vi "PROCESS_CREATION_SCRIPTING.vi"() -> ()   [LabVIEW 2011]
uses:
  Ctl/ClusterDefineNewProcess.ctl
  050 - CONFIG/20 - ExternalProcesses/paramsExternalProcesses.ctl
  Ctl/AppContext.ctl
  Ctl/EnumProcessState.ctl
  Ctl/ClusterProcessCreationScript.ctl
  Ctl/EnumFPOrder.ctl
  <vilib>/event_ctls.llb/eventvkey.ctl
  <vilib>/regexp/Match Regular Expression.xnode
panel:
  in  "discardKey":bool
  in  "Cluster_process":T1={"Process name"="", "viToLaunchInfos"={"File Path Control"=path "", "Timeout"=10.0, "viInitString"="", "State"=enum."Standard"}}
  out "error out":errorcluster
  in  "Test PushButton":bool
  in  "Delete Process PushButton":bool
  in  "Existing processes":i32(listbox)
  in  "Close PushButton":bool
  in  "Create Process PushButton":bool
  # "PROCESS CREATION WIZARD"
  # "Version 1.0"
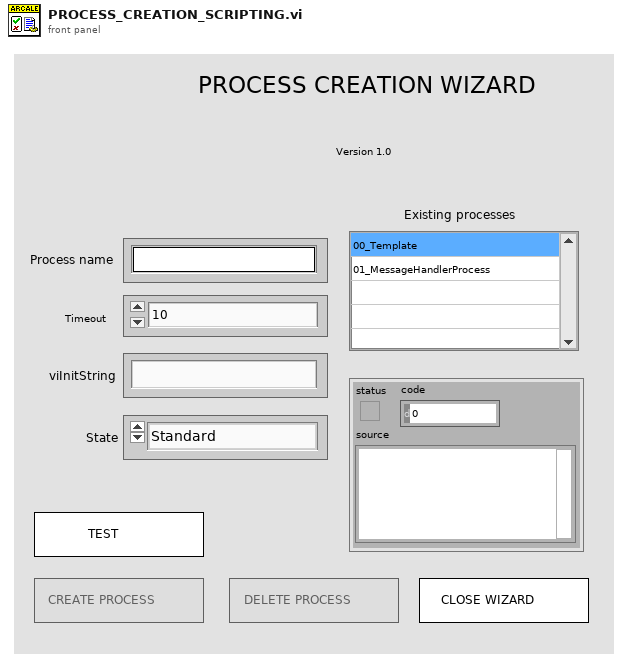
[diagram p1: front panel]
types:
  T1 = typedef "ClusterDefineNewProcess.ctl" = cluster{"Process name":string, "viToLaunchInfos":T2}
  T2 = typedef "paramsExternalProcesses.ctl" = cluster{"File Path Control":path, "Timeout":dbl, "viInitString":string, "State":enum32{"Invalid", "Standard", "Closed", "Hidden", "Minimized", "Maximized"}}
  T3 = enum8{"Enabled", "Disabled", "Disabled and Grayed Out"}
  T4 = typedef "AppContext.ctl" = cluster{"VIRefToProcessTemplate":refnum<vi>, "VIRefToThisVI":refnum<vi>, "ProcessesList":string[], "VIRefToEnumProcess":refnum<vi>, "VIRefTogetProcessViPath":refnum<vi>, "ProcessManagement":cluster{"EnumProcessState":T5, "ProcessName":string, "PathToProcess":path}, "VIRefToSetup":refnum<vi>, "VIRefToStartProcess":refnum<vi>, "ProcessConfig":T2}
  T5 = typedef "EnumProcessState.ctl" = enum16{"Create process", "Delete process"}
  T6 = typedef "ClusterProcessCreationScript.ctl" = cluster{"Variant":variant, "Front Panel Order":T7}
  T7 = typedef "EnumFPOrder.ctl" = enum16{"Test", "Create process", "Delete process", "Close wizard"}
  T8 = typedef "eventvkey.ctl" = enum16{"ASCII", "Enter", "Return", "Shift", "Ctrl", "Alt", "Cmd", "Opt", "Caps", "NumLock", "Clear", "Break", "Up", "Down", "Left", "Right", "Insert", "Delete", "Home", "End", "PageUp", "PageDown", "Escape", "Help", "Pause", "ScrollLock", "F1", "F2", "F3", "F4", "F5", "F6", "F7", "F8", "F9", "F10", "F11", "F12", "F13", "F14", "F15", "F16", "F17", "F18", "F19", "F20", "F21", "F22", "F23", "F24", "Play", "VolumeUp", "VolumeDown", "Mute", "Two Byte Char"}
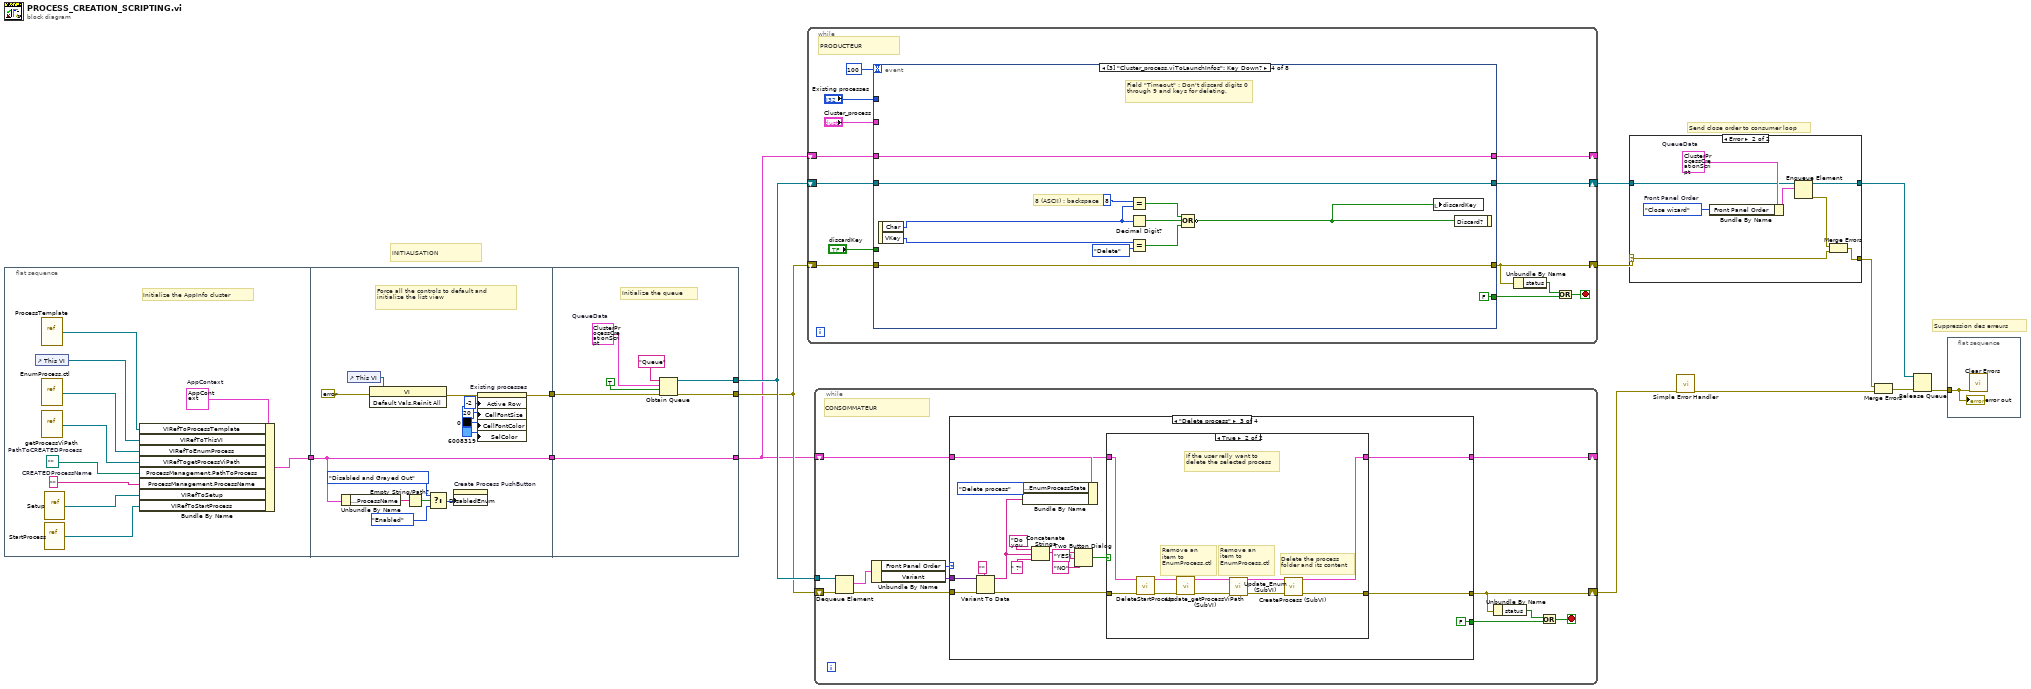
[diagram p0: block diagram]
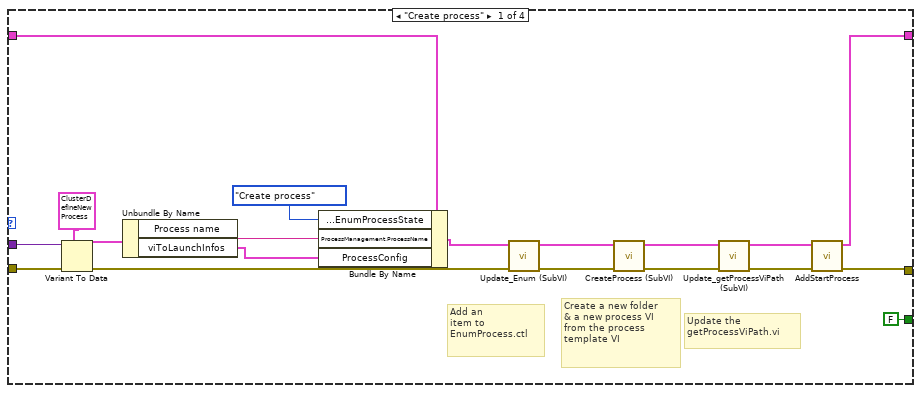
[diagram p3: hidden frame]
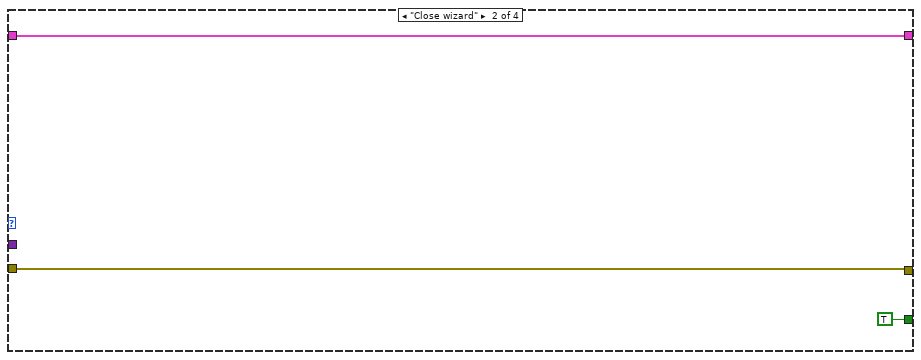
[diagram p4: hidden frame]
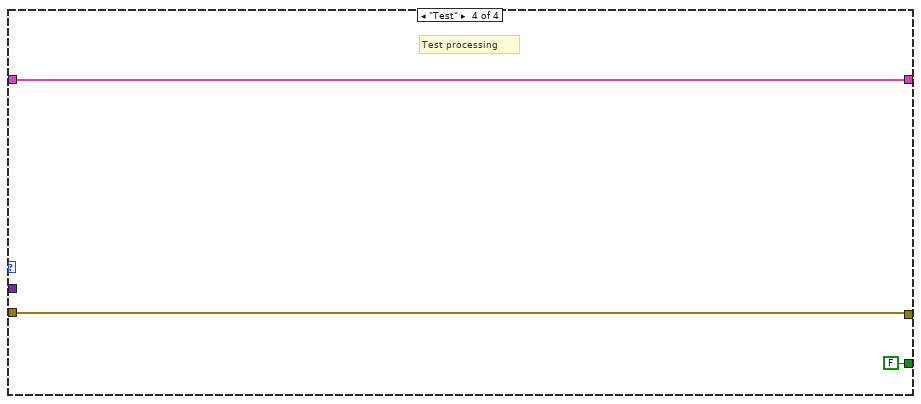
[diagram p6: hidden frame]
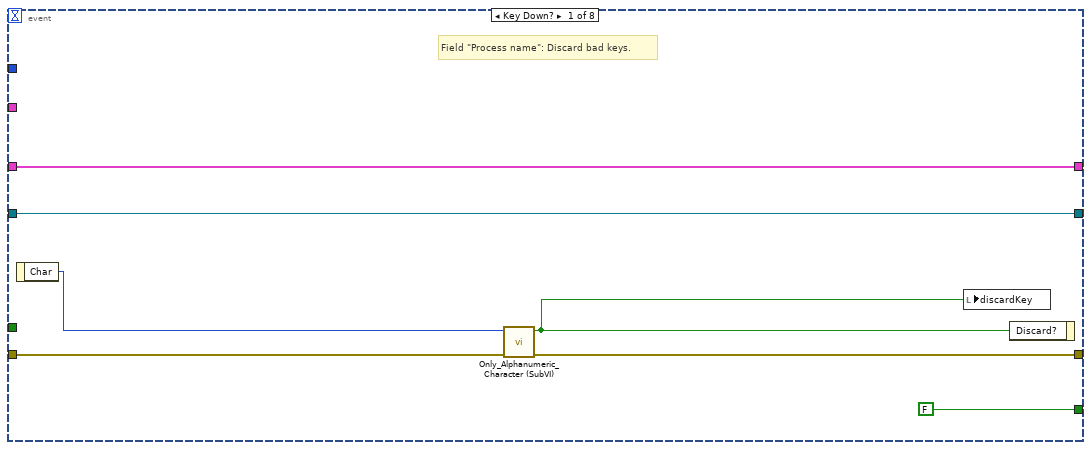
[diagram p7: hidden frame]
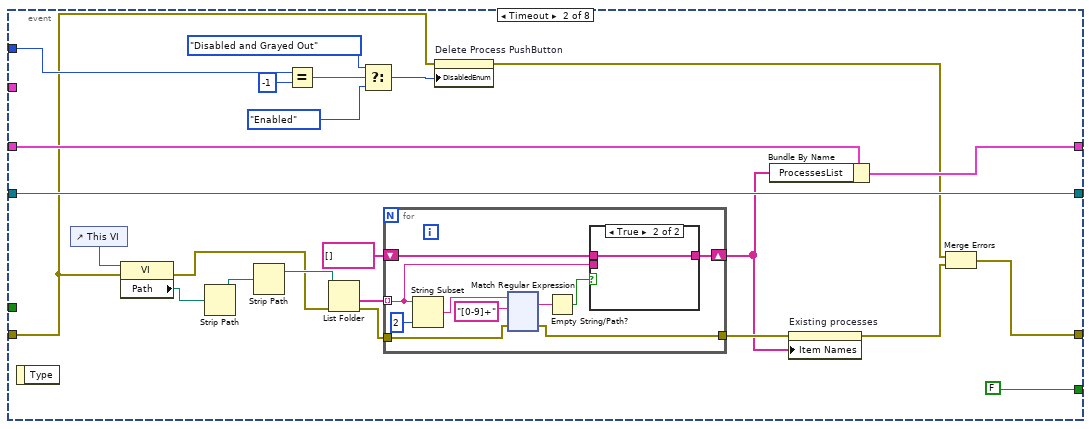
[diagram p8: hidden frame]
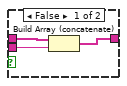
[diagram p9: hidden frame]
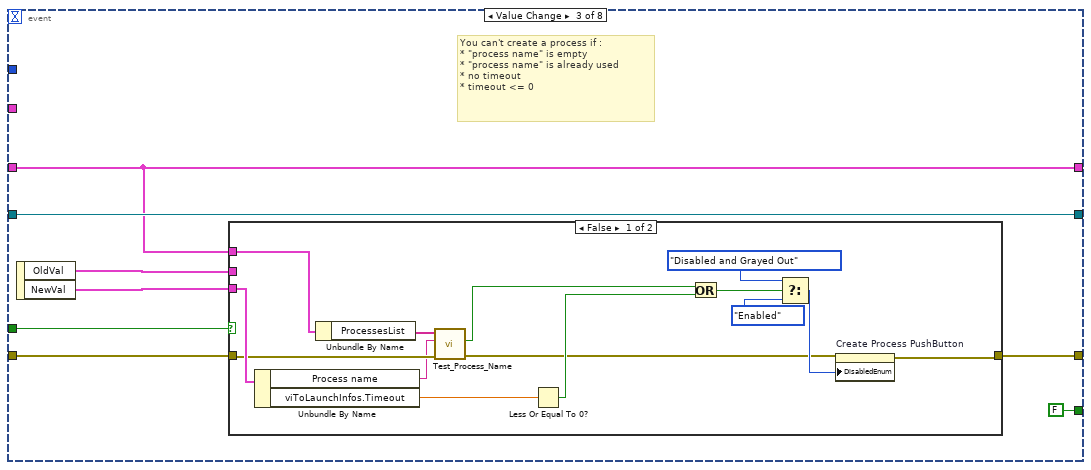
[diagram p10: hidden frame]
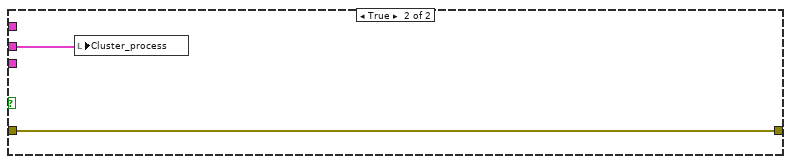
[diagram p11: hidden frame]
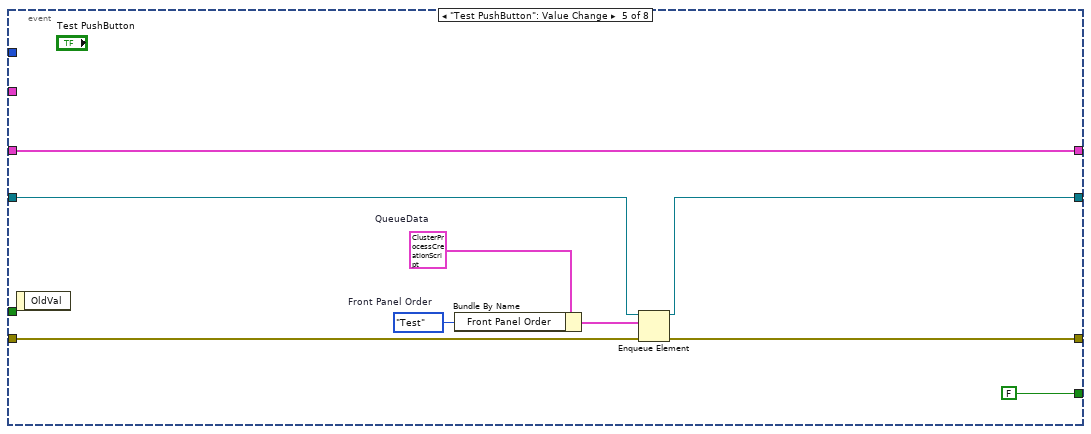
[diagram p12: hidden frame]
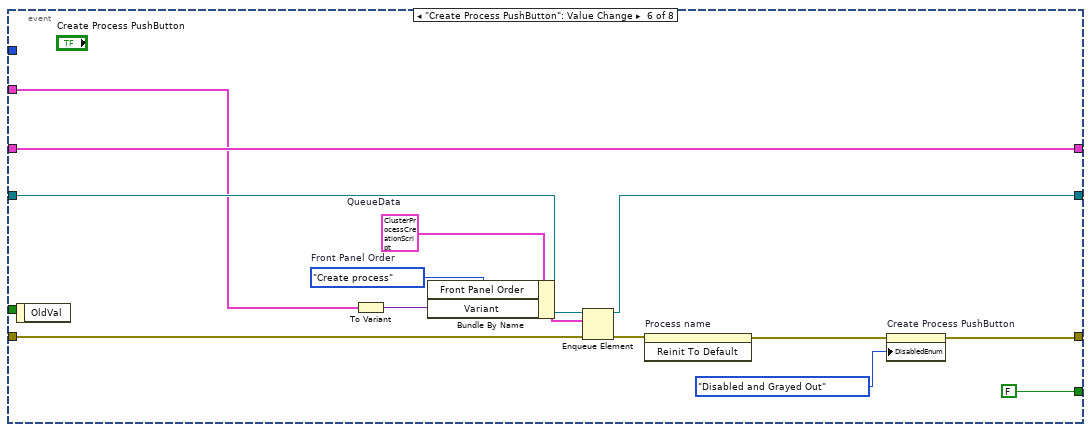
[diagram p13: hidden frame]
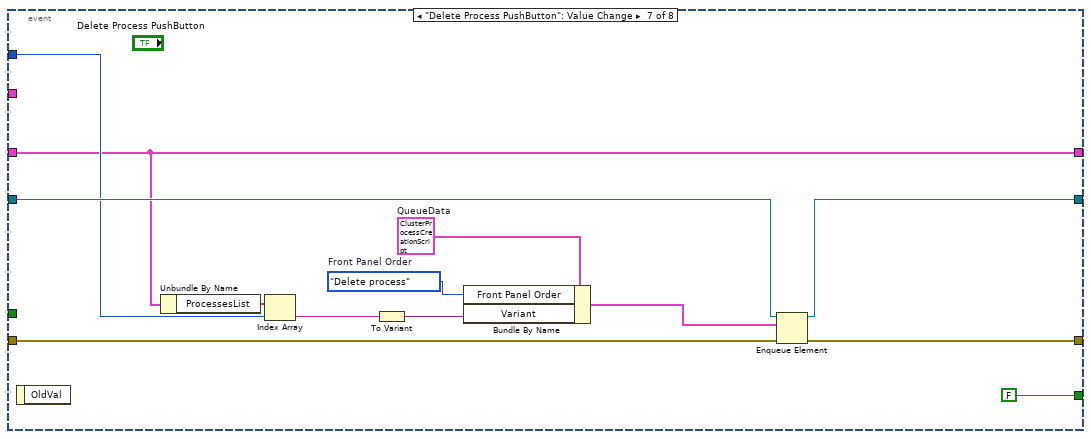
[diagram p14: hidden frame]
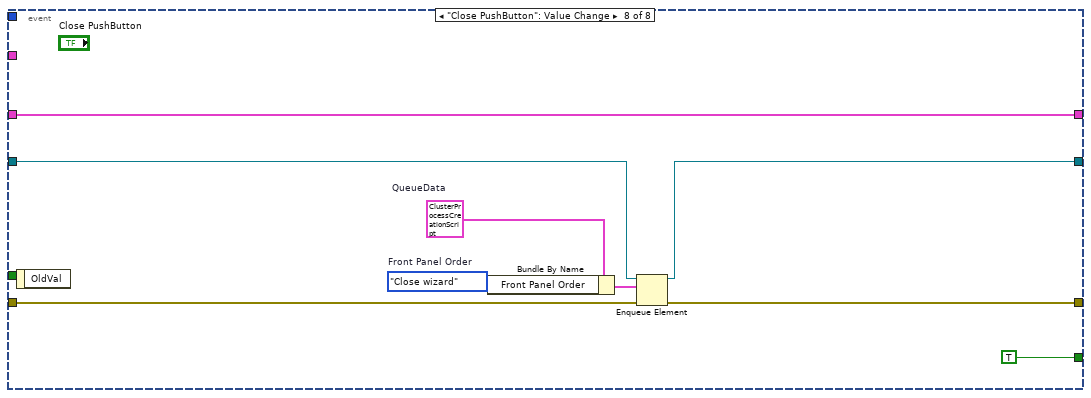
[diagram p15: hidden frame]
diagram:
  # "Send close order to consumer loop"
  # "Suppression des erreurs"
  # "INITIALISATION"
  n1 = flat-sequence {
    tunnel: [w22] -> w8
    tunnel: [w35] -> w10
    tunnel: [w30] -> w9
    tunnel: w8 -> [w30]
    tunnel: [w42] -> w14
    tunnel: [w41] -> w13
    tunnel: w10 -> [w40]
    tunnel: [w39] -> w7
    tunnel: w9 -> [w39]
    frame #0 {
      w17 = T4 {"VIRefToProcessTemplate"=refnum, "VIRefToThisVI"=refnum, "ProcessesList"=[], "VIRefToEnumProcess"=refnum, "VIRefTogetProcessViPath"=refnum, "ProcessManagement"={"EnumProcessState"=enum."Create process", "ProcessName"="", "PathToProcess"=path ""}, "VIRefToSetup"=refnum, "VIRefToStartProcess"=refnum, "ProcessConfig"={"File Path Control"=path "", "Timeout"=0.0, "viInitString"="", "State"=enum."Invalid"}}  # AppContext
      w18 = ""  # CREATEDProcessName
      w19 = path ""  # PathToCREATEDProcess
      # "Initialize the AppInfo cluster"
      n2 = control-ref of="This VI"() -> (w23:refnum<vi>)
      n3 = vi-ref "ProcessTemplate.vi"() -> (w24:refnum<vi>)
      n4 = vi-ref "EnumProcess.ctl"() -> (w21:refnum<vi>)
      n5 = vi-ref "getProcessViPath.vi"() -> (w20:refnum<vi>)
      n6 = vi-ref "StartProcess.vi"() -> (w15:refnum<vi>)
      n7 = vi-ref "Setup.vi"() -> (w16:refnum<vi>)
      n8 = Bundle By Name(cluster=w17, "VIRefToProcessTemplate"=w24, "VIRefToThisVI"=w23, "VIRefToEnumProcess"=w21, "VIRefTogetProcessViPath"=w20, "ProcessManagement.PathToProcess"=w19, "ProcessManagement.ProcessName"=w18, "VIRefToSetup"=w16, "VIRefToStartProcess"=w15) -> (w22:T4)
    }
    frame #1 {
      # "Force all the controls to default and\ninitialize the list view"
      n9 = Unbundle By Name(w30) -> ("ProcessManagement.ProcessName"=w29:string)
      n10 = control-ref of="This VI"() -> (w38:refnum<vi>)
      n11 = invoke class="VI" method="Default Vals.Reinit All"(reference=w38, error in=errorcluster {"status"=FALSE, "code"=0, "source"=""} ("error in (no error)")) -> (error out=w36:errorcluster)  [unwired: 1 in, 2 out]
      n12 = Empty String/Path?(string/path=w29) -> (empty?=w25:bool)
      n13 = Select(t=T3."Disabled and Grayed Out" ("Disabled"), s=w25, f=T3."Enabled") -> (s? t:f=w27:T3)
      n14 = property on="Create Process PushButton" class="Bool"("DisabledEnum"=w27) -> ()  [unwired: 2 in, 2 out]
      n15 = property on="Existing processes" class="LstBox (strict)"(error in=w36, "Active Row"=-2 ("Active Row:Active Row Number"), "CellFontSize"=u32 20 ("Active Row:Cell Font:Size"), "CellFontColor"=u32 0, "SelColor"=u32 6008319) -> (error out=w35:errorcluster)  [unwired: 1 in, 1 out]
    }
    frame #2 {
      w44 = T6 {"Variant"=variant, "Front Panel Order"=enum."Create process"}  # QueueData
      # "Initialize the queue"
      n16 = Obtain Queue(name (unnamed)="Queue", element data type=w44, create if not found? (T)=TRUE, error in (no error)=w40) -> (queue out=w42:refnum<queue>, error out=w41:errorcluster)  [unwired: 1 in, 1 out]
    }
  }
  n17 = while {
    shift-right: [w56] -> w6
    shift-left: w14 -> [w58]
    shift-right: [w49] -> w4
    shift-left: w13 -> [w57]
    shift-right: [w52] -> _
    shift-left: w7 -> [w53]
    stop <- w50 stop-if-true
    # "PRODUCTEUR"
    n18 = event shown="[3] \"Cluster_process.viToLaunchInfos\": Key Down?" {
      selector: _ -> [_ _ _ _ _ _ _ _]
      dyn-events: _ -> [_ _ _ _ _ _ _ _]
      timeout: 100 -> [_ _ _ _ _ _ _ _]
      tunnel: w58 -> [w65 w89 w222 w249 w258 w272 w285 w295]
      tunnel: w57 -> [w62 w69 w219 w250 w257 w270 w284 w293]
      tunnel: [w65 w89 w222 w249 w255 w271 w283 w291] -> w56
      tunnel: [w60 w66 w218 w250 w254 w261 w282 w292] -> w49
      tunnel: "Cluster_process" -> [_ _ _ _ _ w264 _ _]
      tunnel: "Existing processes" -> [_ w70 _ _ _ _ w280 _]
      tunnel: w53 -> [w64 w79 w216 w248 w256 w269 w279 w290]
      tunnel: [w64 w77 w216 w248 w256 w269 w279 w290] -> w52
      tunnel: [FALSE ("y") FALSE ("y") FALSE ("y") FALSE ("y") FALSE ("y") FALSE ("y") FALSE ("y") TRUE ("y")] -> w48
      tunnel: "discardKey" -> [_ _ w217 _ _ _ _ _]
      event Key Down? {
        # "Field \"Process name\": Discard bad keys."
        n19 = event-data() -> ("Char"=w61:i16)  [unwired: 1 in]
        n20 = call "Only_Alphanumeric_Character (SubVI).vi"("error in (no error)"=w62, "Character"=w61) -> ("error out (no error)"=w60:errorcluster, "Discard character taped"=w59:bool)  [unwired: 8 in]
        n21 = local write "discardKey"(w59) -> ()
        n22 = event-data("Discard?"=w59) -> ()  [unwired: 1 in, 1 out]
      }
      event Timeout {
        n23 = event-data() -> ()  [unwired: 1 in, 1 out]
        n24 = control-ref of="This VI"() -> (w86:refnum<vi>)
        n25 = property class="VI"(reference=w86, error in=w69) -> (error out=w84:errorcluster, "Path"=w85:path)  [unwired: 1 out]
        n26 = Strip Path(path=w85) -> (stripped path=w88:path)  [unwired: 1 out]
        n27 = Strip Path(path=w88) -> (stripped path=w87:path)  [unwired: 1 out]
        n28 = Equal?(x=w70, y=-1) -> (x = y?=w74:bool)
        n29 = List Folder(path=w87, error in=w84) -> (folder names=w83:string[], error out=w82:errorcluster)  [unwired: 2 in, 2 out]
        n30 = Select(t=T3."Disabled and Grayed Out" ("Disabled"), s=w74, f=T3."Enabled") -> (s? t:f=w71:T3)
        n31 = for {
          tunnel: w83 -> [w91] mode=indexing
          tunnel: w82 -> [w97]
          shift-right: [w95] -> w78
          shift-left: string[] [] -> [w93]
          tunnel: [w90] -> w80
          n32 = String Subset(string=w91, length (rest)=2 ("length (rest)")) -> (substring=w92:string)  [unwired: 1 in]
          n33 = xnode "Match Regular Expression"("input string"=w92, "regular expression"="[0-9]+", "error in"=w97) -> ("whole match"=w94:string, "error out"=w90:errorcluster)  [unwired: 3 in, 3 out]
          n34 = Empty String/Path?(string/path=w94) -> (empty?=w96:bool)
          n35 = case shown="True" w96 {
            tunnel: [w102 w103] -> w95
            tunnel: w91 -> [w101 _]
            tunnel: w93 -> [w100 w103]
            frame False {
              n36 = Build Array (concatenate)(w100, w101) -> (w102:string[])
            }
            frame True {
            }
          }
        }
        n37 = property on="Delete Process PushButton" class="Bool"(error in=w69, "DisabledEnum"=w71) -> (error out=w68:errorcluster)  [unwired: 1 in, 1 out]
        n38 = Bundle By Name(cluster=w79, "ProcessesList"=w78) -> (w77:T4)
        n39 = property on="Existing processes" class="LstBox (strict)"(error in=w80, "Item Names"=w78) -> (error out=w67:errorcluster)  [unwired: 1 in, 1 out]
        n40 = Merge Errors(w68, w67) -> (w66:errorcluster)
      }
      event Value Change {
        # "You can't create a process if :\n* \"process name\" is empty\n* \"process name\" is already used\n* no timeout\n* timeout <= 0"
        n41 = event-data() -> ("OldVal"=w220:T1, "NewVal"=w215:T1)  [unwired: 1 in]
        n42 = case shown="False" w217 {
          tunnel: w220 -> [_ w238]
          tunnel: w219 -> [w228 w237]
          tunnel: [w227 w237] -> w218
          tunnel: w216 -> [w230 _]
          tunnel: w215 -> [w229 _]
          frame False {
            n43 = Unbundle By Name(w229) -> ("Process name"=w226:string, "viToLaunchInfos.Timeout"=w225:dbl)
            n44 = Unbundle By Name(w230) -> ("ProcessesList"=w234:string[])
            n45 = call "Test_Process_Name.vi"("error in (no error)"=w228, "ProcessName"=w226, "ProcessesList"=w234) -> ("error out"=w223:errorcluster, "incorrectName"=w235:bool)  [unwired: 7 in]
            n46 = Less Or Equal To 0?(x=w225) -> (x <= 0?=w224:bool)
            n47 = Or(x=w235, y=w224) -> (x .or. y?=w236:bool)
            n48 = Select(t=T3."Disabled and Grayed Out" ("Disabled"), s=w236, f=T3."Enabled") -> (s? t:f=w231:T3)
            n49 = property on="Create Process PushButton" class="Bool"(error in=w223, "DisabledEnum"=w231) -> (error out=w227:errorcluster)  [unwired: 1 in, 1 out]
          }
          frame True {
            n50 = local write "Cluster_process"(w238) -> ()
          }
        }
      }
      event Key Down? {
        # "8 (ASCII) : backspace"
        # "Field \"Timeout\" : Don't discard digits 0 through 9 and keys for deleting."
        n51 = event-data() -> ("Char"=w244:i16, "VKey"=w246:T8)  [unwired: 1 in]
        n52 = Equal?(x=i16 8, y=w244) -> (x = y?=w242:bool)
        n53 = Decimal Digit?(1:w244) -> (0:w241:bool)
        n54 = Equal?(x=w246, y=eventvkey."Delete") -> (x = y?=w240:bool)
        n55 = Compound Arithmetic op=OR(w242, w241, w240) -> (invert w239:bool)
        n56 = local write "discardKey"(w239) -> ()
        n57 = event-data("Discard?"=w239) -> ()  [unwired: 1 in, 1 out]
      }
      event "Test PushButton": Value Change {
        w252 = EnumFPOrder."Test"  # Front Panel Order
        w253 = T6 {"Variant"=variant, "Front Panel Order"=enum."Create process"}  # QueueData
        n58 = event-data() -> ()  [unwired: 1 in, 1 out]
        n59 = Bundle By Name(cluster=w253, "Front Panel Order"=w252) -> (w259:T6)
        n60 = Enqueue Element(queue=w258, element=w259, error in (no error)=w257) -> (queue out=w255:refnum<queue>, error out=w254:errorcluster)  [unwired: 1 in, 1 out]
      }
      event "Create Process PushButton": Value Change {
        w267 = T6 {"Variant"=variant, "Front Panel Order"=enum."Create process"}  # QueueData
        w268 = EnumFPOrder."Create process"  # Front Panel Order
        n61 = event-data() -> ()  [unwired: 1 in, 1 out]
        n62 = To Variant(anything=w264) -> (Variant=w263:variant)
        n63 = Bundle By Name(cluster=w267, "Front Panel Order"=w268, "Variant"=w263) -> (w273:T6)
        n64 = Enqueue Element(queue=w272, element=w273, error in (no error)=w270) -> (queue out=w271:refnum<queue>, error out=w265:errorcluster)  [unwired: 1 in, 1 out]
        n65 = invoke on="Process name" class="Str" method="Reinit To Default"(error in=w265) -> (error out=w262:errorcluster)  [unwired: 2 in, 2 out]
        n66 = property on="Create Process PushButton" class="Bool"(error in=w262, "DisabledEnum"=T3."Disabled and Grayed Out" ("Disabled")) -> (error out=w261:errorcluster)  [unwired: 1 in, 1 out]
      }
      event "Delete Process PushButton": Value Change {
        w277 = T6 {"Variant"=variant, "Front Panel Order"=enum."Create process"}  # QueueData
        w278 = EnumFPOrder."Delete process"  # Front Panel Order
        n67 = event-data() -> ()  [unwired: 1 in, 1 out]
        n68 = Unbundle By Name(w279) -> ("ProcessesList"=w281:string[])
        n69 = Index Array(array=w281, index=w280) -> (element=w275:string)
        n70 = To Variant(anything=w275) -> (Variant=w274:variant)
        n71 = Bundle By Name(cluster=w277, "Front Panel Order"=w278, "Variant"=w274) -> (w286:T6)
        n72 = Enqueue Element(queue=w285, element=w286, error in (no error)=w284) -> (queue out=w283:refnum<queue>, error out=w282:errorcluster)  [unwired: 1 in, 1 out]
      }
      event "Close PushButton": Value Change {
        w288 = EnumFPOrder."Close wizard"  # Front Panel Order
        w289 = T6 {"Variant"=variant, "Front Panel Order"=enum."Create process"}  # QueueData
        n73 = event-data() -> ()  [unwired: 1 in, 1 out]
        n74 = Bundle By Name(cluster=w289, "Front Panel Order"=w288) -> (w294:T6)
        n75 = Enqueue Element(queue=w295, element=w294, error in (no error)=w293) -> (queue out=w291:refnum<queue>, error out=w292:errorcluster)  [unwired: 1 in, 1 out]
      }
    }
    n76 = Unbundle By Name(w49) -> ("status"=w51:bool)
    n77 = Or(x=w51, y=w48) -> (x .or. y?=w50:bool)
  }
  n78 = while {
    tunnel: w14 -> [w307]
    shift-right: [w298] -> w2
    shift-left: w13 -> [w306]
    shift-right: [w300] -> _
    shift-left: w7 -> [w303]
    stop <- w296 stop-if-true
    # "CONSOMMATEUR"
    n79 = Dequeue Element(queue=w307, error in (no error)=w306) -> (element=w305:T6, error out=w301:errorcluster)  [unwired: 1 in, 2 out]
    n80 = Unbundle By Name(w305) -> ("Front Panel Order"=w304:T7, "Variant"=w302:variant)
    n81 = case shown="\"Delete process\"" w304 {
      tunnel: [w312 w328 w338 w360] -> w298
      tunnel: w303 -> [w323 w329 w334 w359]
      tunnel: w302 -> [w325 _ w336 _]
      tunnel: w301 -> [w324 w328 w335 w360]
      tunnel: [w311 w329 w330 w359] -> w300
      tunnel: [FALSE TRUE FALSE FALSE] -> w299
      frame "Create process" {
        # "Update the\ngetProcessViPath.vi"
        # "Create a new folder\n& a new process VI\nfrom the process \ntemplate VI"
        # "Add an\nitem to\nEnumProcess.ctl"
        n82 = Variant To Data(error in=w324, type=T1 {"Process name"="", "viToLaunchInfos"={"File Path Control"=path "", "Timeout"=0.0, "viInitString"="", "State"=enum."Invalid"}} ("Cluster_process"), Variant=w325) -> (data=w316:T1, error out=w308:errorcluster)
        n83 = Unbundle By Name(w316) -> ("Process name"=w315:string, "viToLaunchInfos"=w309:T2)
        n84 = Bundle By Name(cluster=w323, "ProcessManagement.EnumProcessState"=EnumProcessState."Create process", "ProcessManagement.ProcessName"=w315, "ProcessConfig"=w309) -> (w322:T4)
        n85 = call "Update_Enum (SubVI).vi"("error in"=w308, "AppContext in"=w322) -> ("error out"=w326:errorcluster, "AppContext out"=w320:T4)  [unwired: 8 in]
        n86 = call "CreateProcess (SubVI).vi"("error in"=w326, "AppContext in"=w320) -> ("error out"=w321:errorcluster, "AppContext out"=w319:T4)  [unwired: 8 in]
        n87 = call "Update_getProcessViPath (SubVI).vi"("error in (no error)"=w321, "AppContext in"=w319) -> ("error out"=w313:errorcluster, "AppContext out"=w314:T4)  [unwired: 7 in]
        n88 = call "AddStartProcess.vi"("error in (no error)"=w313, "AppContextIn"=w314) -> ("error out"=w312:errorcluster, "AppContextOut"=w311:T4)  [unwired: 8 in]
      }
      frame "Close wizard" {
      }
      frame "Delete process" {
        n89 = Variant To Data(error in=w335, type="", Variant=w336) -> (data=w331:string, error out=w340:errorcluster)
        n90 = Bundle By Name(cluster=w334, "ProcessManagement.EnumProcessState"=EnumProcessState."Delete process", "ProcessManagement.ProcessName"=w331) -> (w332:T4)
        n91 = Concatenate Strings("Do you really want to delete the following process " ("string"), w331, " ?" ("string")) -> (w343:string)
        n92 = Two Button Dialog(message=w343, 1:"NO" ("F button name (\"Cancel\")"), 2:"YES" ("T button name (\"OK\")")) -> (T button?=w339:bool)
        n93 = case shown="True" w339 {
          tunnel: w340 -> [w348 w351]
          tunnel: [w348 w357] -> w338
          tunnel: w332 -> [w347 w350]
          tunnel: [w347 w358] -> w330
          frame False {
          }
          frame True {
            # "Remove an\nitem to\nEnumProcess.ctl"
            # "Remove an\nitem to\nEnumProcess.ctl"
            # "Delete the process\nfolder and its content"
            # "If the user relly want to\ndelete the selected process"
            n94 = call "DeleteStartProcess.vi"("error in (no error)"=w351, "AppContextIn"=w350) -> ("error out"=w352:errorcluster, "AppContextOut"=w349:T4)  [unwired: 8 in]
            n95 = call "Update_getProcessViPath (SubVI).vi"("error in (no error)"=w352, "AppContext in"=w349) -> ("error out"=w353:errorcluster, "AppContext out"=w356:T4)  [unwired: 7 in]
            n96 = call "Update_Enum (SubVI).vi"("error in"=w353, "AppContext in"=w356) -> ("error out"=w354:errorcluster, "AppContext out"=w355:T4)  [unwired: 8 in]
            n97 = call "CreateProcess (SubVI).vi"("error in"=w354, "AppContext in"=w355) -> ("error out"=w357:errorcluster, "AppContext out"=w358:T4)  [unwired: 8 in]
          }
        }
      }
      frame "Test" {
        # "Test processing"
      }
    }
    n98 = Unbundle By Name(w298) -> ("status"=w297:bool)
    n99 = Or(x=w297, y=w299) -> (x .or. y?=w296:bool)
  }
  n100 = case shown="Error" w4 {
    selector: w4 -> [w362 w365]
    tunnel: w6 -> [w363 w368]
    tunnel: [w363 w367] -> w5
    tunnel: [w362 w364] -> w3
    frame No Error {
    }
    frame Error {
      w370 = T6 {"Variant"=variant, "Front Panel Order"=enum."Create process"}  # QueueData
      w371 = EnumFPOrder."Close wizard"  # Front Panel Order
      n101 = Bundle By Name(cluster=w370, "Front Panel Order"=w371) -> (w369:T6)
      n102 = Enqueue Element(queue=w368, element=w369) -> (queue out=w367:refnum<queue>, error out=w366:errorcluster)  [unwired: 2 in, 1 out]
      n103 = Merge Errors(w366, w365) -> (w364:errorcluster)
    }
  }
  n104 = call <vilib>:"Simple Error Handler.vi"("error in (no error)"=w2) -> ("error out"=w1:errorcluster)  [unwired: 4 in, 4 out]
  n105 = Merge Errors(w3, w1) -> (w12:errorcluster)
  n106 = Release Queue(queue=w5, error in (no error)=w12) -> (error out=w11:errorcluster)  [unwired: 1 in, 2 out]
  n107 = flat-sequence {
    tunnel: w11 -> [w372]
    frame #0 {
      n108 = call <vilib>:"Clear Errors.vi"("error in (no error)"=w372) -> ()  [unwired: 6 in, 1 out]
      "error out" <- w372
    }
  }
